vi "PH_PILS.vis PreAmpEnablingKnob.vi"(0 "i ref in":refnum<vi>, 5 "error IO":errorcluster) -> (14 "i ref out":refnum<vi>, 19 "error out":errorcluster)   [LabVIEW 2014, in "PH_PILS.lvlib"]
uses:
  PH_PILS.lvlib
  PH_Basics/PH_SystemInformation/PH_SystemInformation.lvlib
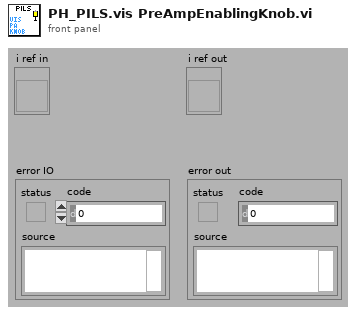
[diagram p1: front panel]
types:
  T1 = typedef "PH_PILS.lvlib/PH_PILS.i attribute.ctl" = cluster{"Boolean":cluster{"GUI Ref":refnum<vi>, "Status":i32}[], "GUI Refs Exp. Shutters":cluster{"1":refnum<vi>, "2":refnum<vi>, "3":refnum<vi>, "4":refnum<vi>}, "Tristate2Run GUI Refs":refnum<vi>[], "EO-Likes":cluster{"GUI Ref":refnum<vi>, "Status":i32}[], "Operation Mode":cluster{"Operation Mode":T2, "GUI":cluster{"Ref State":refnum<vi>, "Ref":refnum<vi>}, "Servicemode":cluster{"Tagname":string, "Status":i32}, "Labormode":cluster{"Tagname":string, "Status":i32}, "Searchmode":cluster{"Tagname":string, "Status":i32}, "Shotmode":cluster{"Tagname":string, "Status":i32}}, "Submode":cluster{"Submode":T3, "GUI":cluster{"Ref State":refnum<vi>, "Ref":refnum<vi>}, "Submode":cluster{"Tagname":string, "Status":i32}}, "Experiment":cluster{"Experiment":enum16{"unknown", "intern", "4 (Z6)", "3", "2", "1"}, "GUI":cluster{"Ref State":refnum<vi>, "Ref":refnum<vi>}, "intern":cluster{"Tagname":string, "Status":i32}, "Exp 4":cluster{"Tagname":string, "Status":i32}, "Exp 3":cluster{"Tagname":string, "Status":i32}, "Exp 2":cluster{"Tagname":string, "Status":i32}, "Exp 1":cluster{"Tagname":string, "Status":i32}}, "TristateNormal":cluster{"GUI Ref":refnum<vi>, "Status":i32}[], "Door Tags":cluster{"GUI Ref":refnum<vi>, "Status":i32}[], "GUIlessTags":cluster{"Name":string, "Status":i32}[], "Beamline GUI Refs":refnum<vi>[], "Special Boolean":cluster{"GUI Ref":refnum<vi>, "Status":i32}[], "Laserpower":cluster{"GUI Ref":refnum<vi>, "Status":i32}[], "Shutter":cluster{"GUI Ref":refnum<vi>, "Status":i32}[], "Tristate EO Like":cluster{"GUI Ref":refnum<vi>, "Status":i32}[], "PP":cluster{"GUI Ref":refnum<vi>, "Status":i32, "Head Ref":refnum<vi>, "Slider Ref":refnum<vi>}[], "Switch Knobs":cluster{"GUI Ref":refnum<vi>, "Status":i32}[], "Latch Knob GUI Refs":refnum<vi>[], "FailureCounter":i32, "Enabled Status":cluster{"Laser":i32, "PreAmp":i32, "MainAmp":i32}, "Mercury":refnum<vi>, "Instance Rods":string, "Logfile":path, "Beckhoff-Instance Internal":string, "Beckhoff-Instance External":string, "Enabling Rights":cluster{"Name":string, "Password":string, "PA?":bool, "MA?":bool, "Exp?":bool}[]}
  T2 = typedef "PH_PILS.lvlib/PH_PILS.Operation Mode.ctl" = enum16{"unknown", "Service", "Labor", "Search", "Shot"}
  T3 = typedef "PH_PILS.lvlib/PH_PILS.Submode.ctl" = enum16{"unknown", "HV-Normal", "HV-Test"}
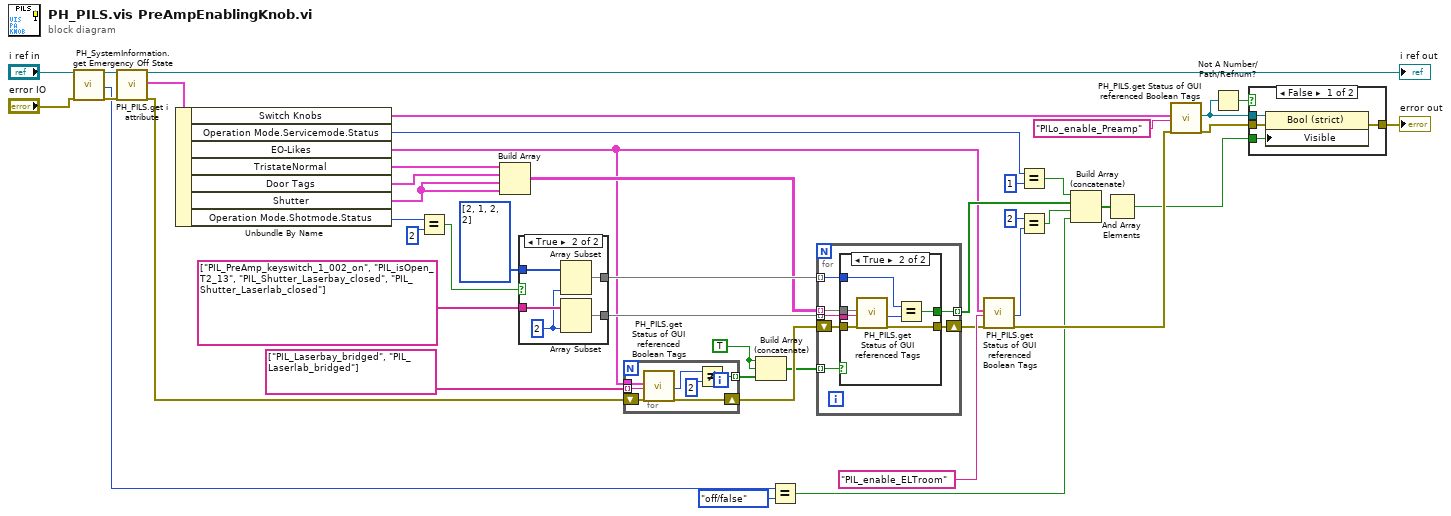
[diagram p0: block diagram]
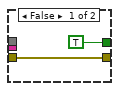
[diagram p4: hidden frame]
diagram:
  w2 = TRUE
  n1 = call "PH_SystemInformation.get Emergency Off State.vi"("i ref in"="i ref in", "error in (no error)"="error IO") -> ("i ref out"=w12:refnum<vi>, "Emergency Off State"=w11:enum16{"no info", "off/false", "Alarm"}, "error out"=w14:errorcluster)  [unwired: 15 in]
  n2 = call "PH_PILS.get i attribute.vi"("i ref in"=w12, "error in (no error)"=w14) -> ("i ref out"=→"i ref out":refnum<vi>, "i attribute"=w43:T1, "error out"=w8:errorcluster)  [unwired: 15 in]
  n3 = Unbundle By Name(w43) -> ("Switch Knobs"=w42:cluster{"GUI Ref":refnum<vi>, "Status":i32}[], "Operation Mode.Servicemode.Status"=w32:i32, "EO-Likes"=w5:cluster{"GUI Ref":refnum<vi>, "Status":i32}[], "TristateNormal"=w36:cluster{"GUI Ref":refnum<vi>, "Status":i32}[], "Door Tags"=w35:cluster{"GUI Ref":refnum<vi>, "Status":i32}[], "Shutter"=w34:cluster{"GUI Ref":refnum<vi>, "Status":i32}[], "Operation Mode.Shotmode.Status"=w24:i32)
  n4 = Equal?(x=w24, y=2) -> (x = y?=w28:bool)
  n5 = Build Array(w36, w35, w34, w34) -> (w6:cluster{"GUI Ref":refnum<vi>, "Status":i32}[][])
  n6 = case shown="True" w28 {
    tunnel: string[] ["PIL_PreAmp_keyswitch_1_002_on", "PIL_isOpen_T2_13", "PIL_Shutter_Laserbay_closed", "PIL_Shutter_Laserlab_closed"] -> [w47 w52]
    tunnel: i32[] [2, 1, 2, 2] -> [w46 w51]
    tunnel: [w47 w49] -> w26
    tunnel: [w46 w48] -> w25
    frame False {
    }
    frame True {
      w50 = 2 ("length")
      n7 = Array Subset(array=w51, length=w50) -> (w48:i32[])  [unwired: 1 in]
      n8 = Array Subset(array=w52, length=w50) -> (w49:string[])  [unwired: 1 in]
    }
  }
  n9 = for {
    shift-right: [w58] -> w7
    shift-left: w8 -> [w59]
    tunnel: w5 -> [w57]
    tunnel: string[] ["PIL_Laserbay_bridged", "PIL_Laserlab_bridged"] -> [w56] mode=indexing
    tunnel: [w53] -> w3 mode=indexing
    n10 = call "PH_PILS.get Status of GUI referenced Boolean Tags.vi"("Tags"=w57, "Tagname"=w56, "error in"=w59) -> ("Status"=w55:i32, "error out"=w58:errorcluster)  [unwired: 13 in, 2 out]
    n11 = Not Equal?(x=w55, y=2) -> (x != y?=w53:bool)
  }
  n12 = Build Array (concatenate)(w2, w2, w3) -> (w1:bool[])
  n13 = Equal?(x=w11, y=enum16{"no info", "off/false", "Alarm"}."off/false") -> (x = y?=w9:bool)
  n14 = for {
    tunnel: w26 -> [w66] mode=indexing
    shift-right: [w65] -> w23
    shift-left: w7 -> [w64]
    tunnel: w6 -> [w63] mode=indexing
    tunnel: w25 -> [w61] mode=indexing
    tunnel: [w62] -> w20 mode=indexing
    tunnel: w1 -> [w60] mode=indexing
    n15 = case shown="True" w60 {
      tunnel: w66 -> [_ w75]
      tunnel: [w67 w74] -> w65
      tunnel: w64 -> [w67 w73]
      tunnel: w63 -> [_ w72]
      tunnel: [TRUE w71] -> w62
      tunnel: w61 -> [_ w70]
      frame False {
      }
      frame True {
        n16 = call "PH_PILS.get Status of GUI referenced Tags.vi"("Tags"=w72, "Tagname"=w75, "error in"=w73) -> ("Status"=w69:i32, "error out"=w74:errorcluster)  [unwired: 13 in, 2 out]
        n17 = Equal?(x=w70, y=w69) -> (x = y?=w71:bool)
      }
    }
  }
  n18 = call "PH_PILS.get Status of GUI referenced Boolean Tags.vi"("Tags"=w5, "Tagname"="PIL_enable_ELTroom", "error in"=w23) -> ("Status"=w18:i32, "error out"=w22:errorcluster)  [unwired: 13 in, 2 out]
  n19 = Equal?(x=w32, y=1) -> (x = y?=w21:bool)
  n20 = Equal?(x=2 ("y"), y=w18) -> (x = y?=w17:bool)
  n21 = Build Array (concatenate)(w21, w20, w17, w9) -> (w16:bool[])
  n22 = And Array Elements(Boolean array=w16) -> (logical AND=w15:bool)
  n23 = call "PH_PILS.get Status of GUI referenced Boolean Tags.vi"("Tags"=w42, "Tagname"="PILo_enable_Preamp", "error in"=w22) -> ("GUI Ref"=w39:refnum<vi>, "error out"=w41:errorcluster)  [unwired: 13 in, 2 out]
  n24 = Not A Number/Path/Refnum?(number/path/refnum=w39) -> (NaN/Path/Refnum?=w40:bool)
  n25 = case shown="False" w40 {
    tunnel: w41 -> [w79 w80]
    tunnel: w39 -> [w78 _]
    tunnel: [w77 w80] -> w38
    tunnel: w15 -> [w76 _]
    frame False {
      n26 = property class="Bool (strict)"(reference=w78, error in=w79, "Visible"=w76) -> (error out=w77:errorcluster)  [unwired: 1 out]
    }
    frame True {
    }
  }
  "error out" <- w38
